vi "Close.vi"(8 "error in (no error)":errorcluster, 11 "MelsecTCP in":refnum<class "Abstract PLC Controler.lvclass">) -> (0 "error out":errorcluster, 3 "MelsecTCP out":refnum<class "Abstract PLC Controler.lvclass">)   [LabVIEW 2020, in "HslCommunication.lvlib" / "Abstract PLC Controler.lvclass"]
uses:
  Abstract PLC Controler.lvclass
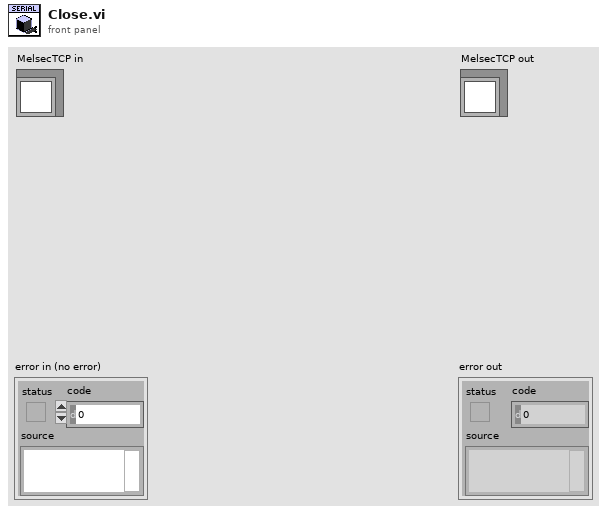
[diagram p1: front panel]
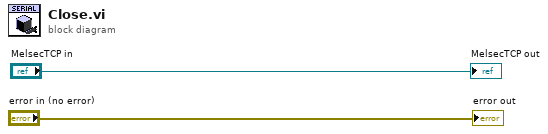
[diagram p0: block diagram]
diagram:
  "error out" <- "error in (no error)"
  "MelsecTCP out" <- "MelsecTCP in"
